vi "Periodic Tasks.vi"(8 "error in":errorcluster) -> ()   [LabVIEW 2020]
doc: "This VI runs in parallel to other tasks. It can contain as many user-defined periodic loops as you need. These can carry out PID or other sorts of timed response."
uses:
  <vilib>/Rock Robotics/WPI/DriverStation/WPI_DriverStationRobotMode2.ctl
  <vilib>/Rock Robotics/WPI/ThirdParty/Phoenix-LabVIEW/Motor Controller/Controls/CTRE_Phoenix_MotorControl_ControlMode.ctl
  <vilib>/Rock Robotics/WPI/Joystick/XBox Axes Indexer.ctl
  <vilib>/Rock Robotics/WPI/Utilities/WPI_GetSetVariantRefNum.vi
  Robot Global Data.vi
  <vilib>/Rock Robotics/Network Tables/NT Read Number.vi
  <vilib>/Rock Robotics/WPI/ThirdParty/Phoenix-LabVIEW/Motor Controller/Get/CTRE_Phoenix_MotorController_GetSelectedSensorData.vi
  <vilib>/Rock Robotics/Network Tables/NT Write Number.vi
  <vilib>/Rock Robotics/WPI/ThirdParty/Phoenix-LabVIEW/Pigeon IMU/CTRE_PigeonIMU_GetYPR.vi
  <vilib>/ptbypt/NI_PtbyPt.lvlib
panel:
  out "Drive Loop Speed":u32=37
  in  "Drive wait":u32=25
  in  "Sensor wait":u32=25
  out "Sensor Loop Speed":u32=26
  in  "Joystick wait":u32=25
  out "Joystick Loop Speed":u32=28
  in  "Rot Pt X":dbl format="%#_13g"
  in  "Rot Pt Y":dbl format="%#_13g"
  out "Robot Centric?":bool
  in  "Slow Drive Speed %":dbl=0.75
  in  "Z-axis rate modifier":dbl=0.7 format="%#_13g"
  out "Go Slow?":bool
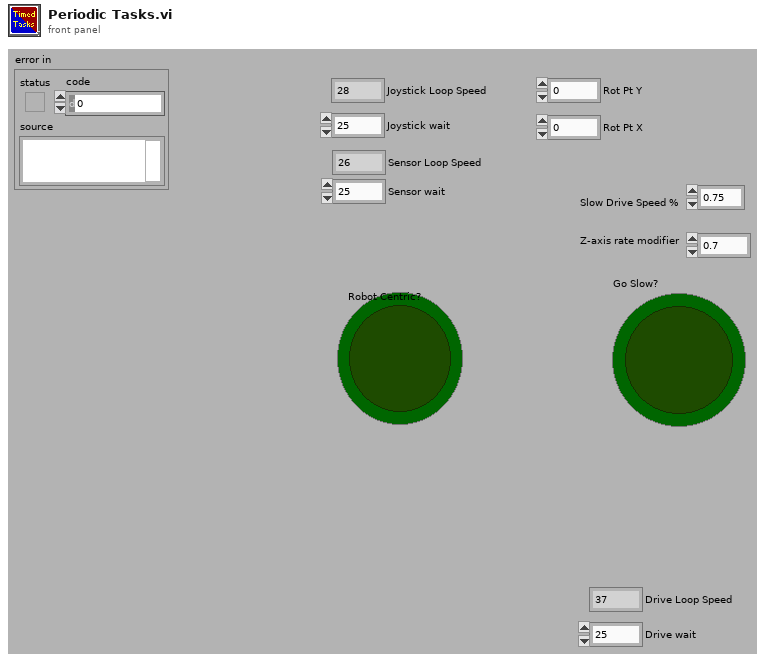
[diagram p1: front panel]
types:
  T1 = typedef "WPI_MotorControlDeviceRef.ctl" = cluster{"DeviceStatus":errorcluster, "Type":T2, "PWM":cluster{"PWM Channel":T3, "DeadBand":T4}, "CAN":cluster{"Device Number":u8, "SetOutput VI Ref":variant, "GetOutput VI Ref":variant, "Enable VI Ref":variant, "Disable VI Ref":variant, "Data":variant}, "Invert":bool, "DIO PWM":cluster{"PWM \"Enable\" Channel":T3, "DIOChannel":T5, "PWM Rate":dbl}}
  T2 = typedef "WPI_MotorControlType.ctl" = enum16{"PWM", "CAN", "DIO PWM"}
  T3 = typedef "FPGA_DIOPWMChannel.ctl" = enum8{"PWM 0", "PWM 1", "PWM 2", "PWM 3", "PWM 4", "PWM 5", "PWM 6", "PWM 7", "PWM 8", "PWM 9", "PWM MXP 0", "PWM MXP 1", "PWM MXP 2", "PWM MXP 3", "PWM MXP 4", "PWM MXP 5", "PWM MXP 6", "PWM MXP 7", "PWM MXP 8", "PWM MXP 9", "Invalid"}
  T4 = typedef "WPI_PWMDeadband.ctl" = cluster{"Name":string, "maxPositivePwm":i32, "minPositivePwm":i32, "centerPwm":i32, "maxNegativePwm":i32, "minNegativePwm":i32, "angularRange":u16}
  T5 = typedef "FPGA_DIOChannel.ctl" = enum8{"DIO 0", "DIO 1", "DIO 2", "DIO 3", "DIO 4", "DIO 5", "DIO 6", "DIO 7", "DIO 8", "DIO 9", "DIO MXP 0", "DIO MXP 1", "DIO MXP 2", "DIO MXP 3", "DIO MXP 4", "DIO MXP 5", "DIO MXP 6", "DIO MXP 7", "DIO MXP 8", "DIO MXP 9", "DIO MXP 10", "DIO MXP 11", "DIO MXP 12", "DIO MXP 13", "DIO MXP 14", "DIO MXP 15", "SPI Port CS1", "SPI Port CS2", "SPI Port CS3", "SPI Port MISO", "SPI Port MOSI", "Invalid"}
  T6 = typedef "WPI_JoystickDevRef.ctl" = cluster{"Device":T7}
  T7 = typedef "WPI_JoystickDeviceEnum.ctl" = enum16{"USB 0", "USB 1", "USB 2", "USB 3", "USB 4", "USB 5"}
  T8 = typedef "XBox Axes Indexer.ctl" = enum16{"Left X", "Left Y", "Left Trigger", "Right Trigger", "Right X", "Right Y"}
  T9 = typedef "WPI_DriverStationRobotMode2.ctl" = enum16{"Autonomous Disabled", "Autonomous Enabled", "Teleop Disabled", "Teleop Enabled", "Disconnected", "Finish", "Test Disabled", "Test Enabled", "Emergency Stopped"}
  T10 = typedef "CTRE_Phoenix_MotorControl_ControlMode.ctl" = u16
  T11 = typedef "CTRE_PigeonIMU_DeviceRef.ctl" = cluster{"DeviceStatus":errorcluster, "Device Number":u8, "Type":T12, "Device ID":u32, "Handle":u64, "UsageFrame":u32, "Library Path":path}
  T12 = typedef "CTRE_PigeonIMU_ConnectionType.ctl" = u32
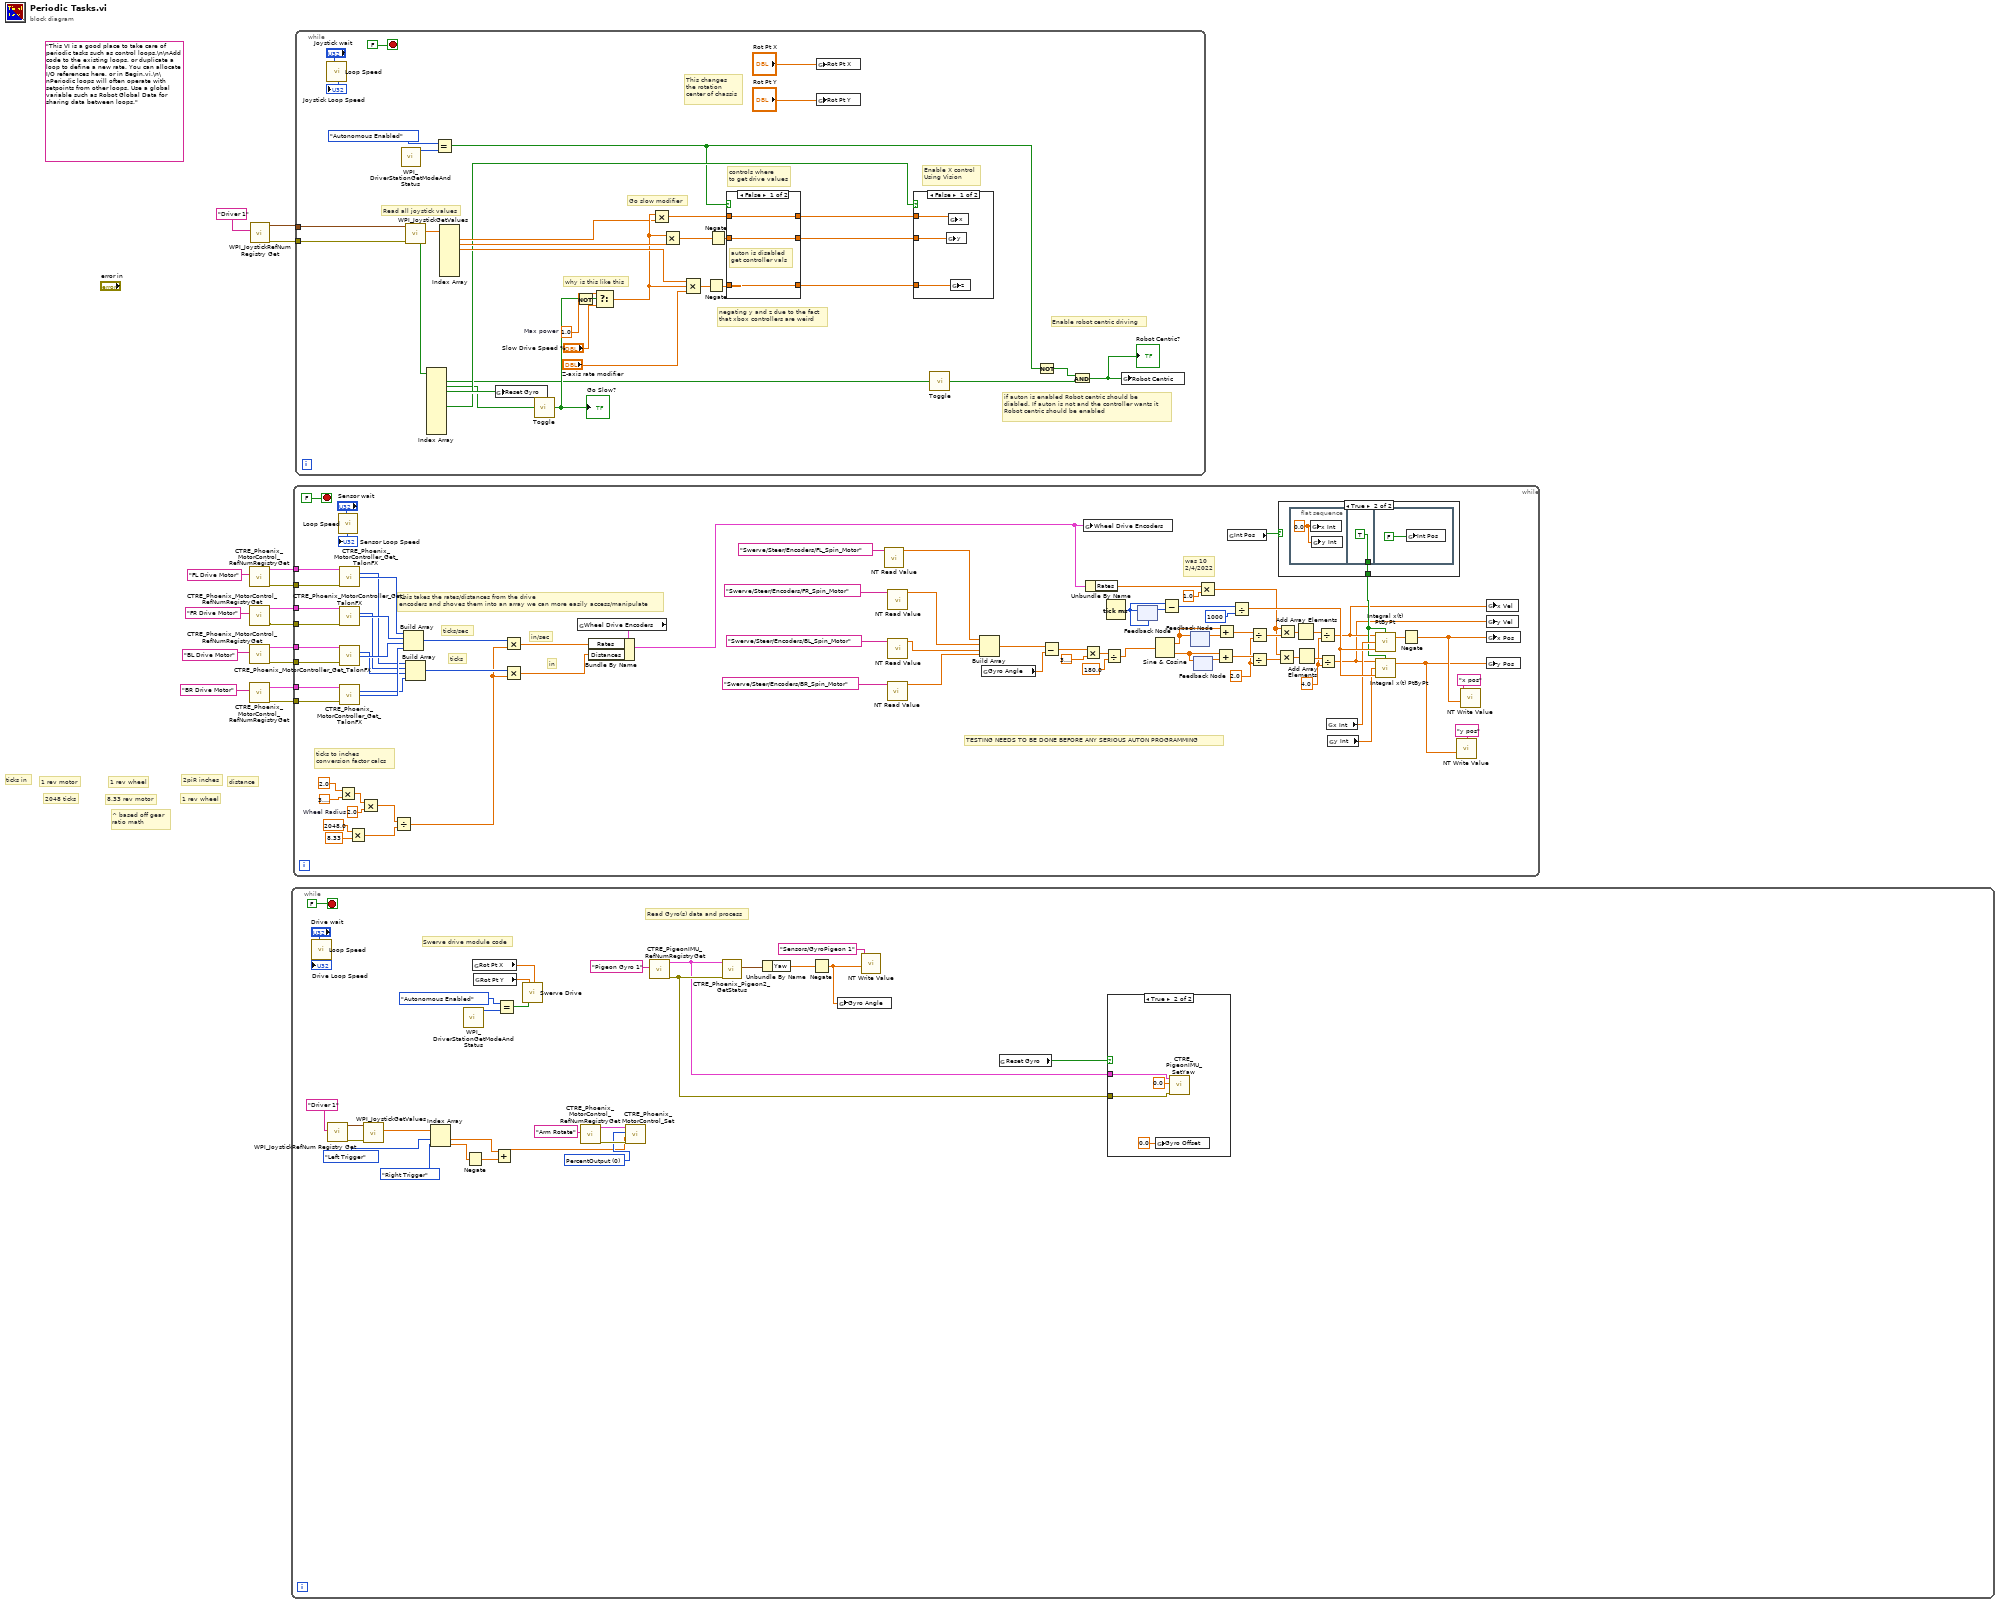
[diagram p0: block diagram]
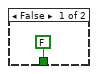
[diagram p3: hidden frame]
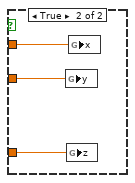
[diagram p4: hidden frame]
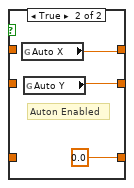
[diagram p5: hidden frame]
diagram:
  (unwired) "This VI is a good place to take care of periodic tasks such as control loops.\n\nAdd code to the existing loops, or duplicate a loop to define a new rate. You can allocate I/O references here, or in Begin.vi.\n\nPeriodic loops will often operate with setpoints from other loops. Use a global variable such as Robot Global Data for sharing data between loops."
  # "^ based off gear \nratio math"
  # "distance"
  # "2piR inches"
  # "1 rev wheel"
  # "1 rev wheel"
  # "8.33 rev motor"
  # "1 rev motor"
  # "2048 ticks"
  # "ticks in"
  n1 = call <vilib>:"CTRE_Phoenix_MotorControl_RefNumRegistryGet.vi"("refnum name"="FL Drive Motor") -> ("error out"=w7:errorcluster, "PhoenixMotorControlDevRef"=w8:T1)  [unwired: 9 in]
  n2 = call <vilib>:"CTRE_Phoenix_MotorControl_RefNumRegistryGet.vi"("refnum name"="FR Drive Motor") -> ("error out"=w5:errorcluster, "PhoenixMotorControlDevRef"=w6:T1)  [unwired: 9 in]
  n3 = call <vilib>:"CTRE_Phoenix_MotorControl_RefNumRegistryGet.vi"("refnum name"="BL Drive Motor") -> ("error out"=w3:errorcluster, "PhoenixMotorControlDevRef"=w4:T1)  [unwired: 9 in]
  n4 = call <vilib>:"CTRE_Phoenix_MotorControl_RefNumRegistryGet.vi"("refnum name"="BR Drive Motor") -> ("error out"=w1:errorcluster, "PhoenixMotorControlDevRef"=w2:T1)  [unwired: 9 in]
  n5 = call <vilib>:"WPI_JoystickRefNum Registry Get.vi"("refnum name"="Driver 1") -> ("error out"=w13:errorcluster, "JoystickDevRef"=w14:T6)  [unwired: 1 in, 8 out]
  n6 = while {
    stop <- FALSE stop-if-true
    w22 = T10 0 items=["PercentOutput"=0, "Position"=1, "Velocity"=2, "Current"=3, "Follower"=5, "MotionProfile"=6, "MotionMagic"=7, "MotionProfileArc"=10, "Disabled"=15] ("Control Mode")
    # "Read Gyro(s) data and process"
    # "Swerve drive module code"
    n7 = call "Loop Speed.vi"("milliseconds to wait"="Drive wait") -> ("Loop Speed"=→"Drive Loop Speed":u32)
    n8 = call <vilib>:"WPI_JoystickRefNum Registry Get.vi"("refnum name"="Driver 1") -> ("error out"=w26:errorcluster, "JoystickDevRef"=w25:T6)  [unwired: 9 in]
    n9 = call <vilib>:"WPI_JoystickGetValues.vi"("error in (no error)"=w26, "JoystickDevRef"=w25) -> ("Axes"=w24:dbl[])  [unwired: 5 in, 4 out]
    n10 = Index Array(array=w24, index #1=XBox_Axes_Indexer."Left Trigger" ("XBox Axes"), index #2=XBox_Axes_Indexer."Right Trigger" ("XBox Axes")) -> (element #1=w18:dbl, element #2=w20:dbl)
    n11 = call <vilib>:"WPI_DriverStationGetModeAndStatus.vi"() -> ("Robot Mode"=w39:T9)  [unwired: 10 in, 1 out]
    n12 = Negate(x=w20) -> (-x=w19:dbl)
    n13 = global read "Robot Global Data.vi" "Rot Pt X"() -> (w41:dbl)
    n14 = global read "Robot Global Data.vi" "Rot Pt Y"() -> (w40:dbl)
    n15 = Add(x=w18, y=w19) -> (x+y=w17:dbl)
    n16 = Equal?(x=WPI_DriverStationRobotMode2."Autonomous Enabled", y=w39) -> (x = y?=w42:bool)
    n17 = call "Swerve Drive.vi"("Rot. Point X"=w41, "Auto Controls"=w42, "Rot. Point Y"=w40) -> ()  [unwired: 9 in]
    n18 = call <vilib>:"CTRE_Phoenix_MotorControl_RefNumRegistryGet.vi"("refnum name"="Arm Rotate") -> ("error out"=w29:errorcluster, "PhoenixMotorControlDevRef"=w28:T1)  [unwired: 9 in]
    n19 = call <vilib>:"CTRE_Phoenix_MotorControl_Set.vi"("error in (no error)"=w29, "Output"=w17, "Control Mode"=w22, "PhoenixMotorControlDevRef"=w28) -> ()  [unwired: 6 in, 2 out]
    n20 = call <vilib>:"CTRE_PigeonIMU_RefNumRegistryGet.vi"("refnum name"="Pigeon Gyro 1") -> ("error out"=w32:errorcluster, "PigeonIMUDevRef"=w31:T11)  [unwired: 9 in]
    n21 = call-poly <vilib>:"CTRE_Phoenix_Pigeon2_GetStatus.vi"("error in (no error)"=w32, "PigeonIMUDevRef"=w31) -> ("Yaw Pitch Roll"=w36:cluster{"Yaw":dbl, "Pitch":dbl, "Roll":dbl})  [unwired: 7 in, 2 out]
    n22 = Unbundle By Name(w36) -> ("Yaw"=w37:dbl)
    n23 = Negate(x=w37) -> (-x=w30:dbl)
    n24 = global write "Robot Global Data.vi" "Gyro Angle"(w30) -> ()
    n25 = call-poly <vilib>:"NT Write Value.vi"("value"=w30, "name"="Sensors/GyroPigeon 1" ("Name")) -> ()  [unwired: 9 in, 1 out]
    n26 = global read "Robot Global Data.vi" "Reset Gyro"() -> (w33:bool)
    n27 = case shown="True" w33 {
      tunnel: w32 -> [_ w47]
      tunnel: w31 -> [_ w46]
      frame False {
      }
      frame True {
        n28 = global write "Robot Global Data.vi" "Gyro Offset"(0.0 ("Gyro Offset")) -> ()
        n29 = call <vilib>:"CTRE_PigeonIMU_SetYaw.vi"("error in (no error)"=w47, "Value"=0.0, "PigeonIMUDevRef"=w46) -> ()  [unwired: 7 in, 2 out]
      }
    }
  }
  n30 = while {
    tunnel: w8 -> [w80]
    tunnel: w7 -> [w79]
    tunnel: w6 -> [w78]
    tunnel: w5 -> [w77]
    tunnel: w4 -> [w76]
    tunnel: w3 -> [w75]
    tunnel: w2 -> [w74]
    tunnel: w1 -> [w73]
    stop <- FALSE stop-if-true
    w66 = 2.0  # Wheel Radius
    w90 = 4.0 ("y")
    w115 = 2.0
    # "TESTING NEEDS TO BE DONE BEFORE ANY SERIOUS AUTON PROGRAMMING"
    # "was 10 \n2/4/2022"
    # "ticks to inches \nconversion factor calcs"
    # "in/sec"
    # "in"
    # "ticks"
    # "ticks/sec"
    # "This takes the rates/distances from the drive \nencoders and shoves them into an array we can more easily access/manipulate"
    n31 = call "Loop Speed.vi"("milliseconds to wait"="Sensor wait") -> ("Loop Speed"=→"Sensor Loop Speed":u32)
    n32 = Multiply(x=2.0, y=3.141592653589793) -> (x*y=w67:dbl)
    n33 = call-poly <vilib>:"CTRE_Phoenix_MotorController_Get_TalonFX.vi"("PhoenixMotorControlDevRef"=w80, "error in"=w79) -> ("Position (Raw Sensor Units)"=w95:i32, "Velocity (Raw Sensor Units per 100 ms)"=w105:i32)  [unwired: 10 in, 2 out]
    n34 = call-poly <vilib>:"CTRE_Phoenix_MotorController_Get_TalonFX.vi"("PhoenixMotorControlDevRef"=w78, "error in"=w77) -> ("Position (Raw Sensor Units)"=w101:i32, "Velocity (Raw Sensor Units per 100 ms)"=w104:i32)  [unwired: 10 in, 2 out]
    n35 = call-poly <vilib>:"CTRE_Phoenix_MotorController_Get_TalonFX.vi"("PhoenixMotorControlDevRef"=w76, "error in"=w75) -> ("Position (Raw Sensor Units)"=w100:i32, "Velocity (Raw Sensor Units per 100 ms)"=w103:i32)  [unwired: 10 in, 2 out]
    n36 = call-poly <vilib>:"CTRE_Phoenix_MotorController_Get_TalonFX.vi"("PhoenixMotorControlDevRef"=w74, "error in"=w73) -> ("Position (Raw Sensor Units)"=w99:i32, "Velocity (Raw Sensor Units per 100 ms)"=w102:i32)  [unwired: 10 in, 2 out]
    n37 = Multiply(x=2048.0, y=8.33) -> (x*y=w64:dbl)
    n38 = Multiply(x=w67, y=w66) -> (x*y=w65:dbl)
    n39 = Divide(x=w65, y=w64) -> (x/y=w59:dbl)
    n40 = Build Array(w105, w104, w103, w102) -> (w60:i32[])
    n41 = Build Array(w95, w101, w100, w99) -> (w62:i32[])
    n42 = Multiply(x=w60, y=w59) -> (x*y=w58:dbl[])
    n43 = Multiply(x=w62, y=w59) -> (x*y=w61:dbl[])
    n44 = global read "Robot Global Data.vi" "Wheel Drive Encoders"() -> (w98:cluster{"Rates":dbl[], "Distances":dbl[]})
    n45 = Bundle By Name(cluster=w98, "Rates"=w58, "Distances"=w61) -> (w72:cluster{"Rates":dbl[], "Distances":dbl[]})
    n46 = call-poly <vilib>:"NT Read Value.vi"("name"="Swerve/Steer/Encoders/FL_Spin_Motor") -> ("value"=w126:dbl)  [unwired: 8 in, 2 out]
    n47 = call-poly <vilib>:"NT Read Value.vi"("name"="Swerve/Steer/Encoders/BR_Spin_Motor") -> ("value"=w123:dbl)  [unwired: 8 in, 2 out]
    n48 = call-poly <vilib>:"NT Read Value.vi"("name"="Swerve/Steer/Encoders/FR_Spin_Motor") -> ("value"=w125:dbl)  [unwired: 8 in, 2 out]
    n49 = call-poly <vilib>:"NT Read Value.vi"("name"="Swerve/Steer/Encoders/BL_Spin_Motor") -> ("value"=w124:dbl)  [unwired: 8 in, 2 out]
    n50 = Build Array(w126, w125, w124, w123) -> (w122:dbl[])
    n51 = global read "Robot Global Data.vi" "Gyro Angle"() -> (w83:dbl)
    n52 = Subtract(x=w122, y=w83) -> (x-y=w88:dbl[])
    n53 = global write "Robot Global Data.vi" "Wheel Drive Encoders"(w72) -> ()
    n54 = Multiply(x=w88, y=3.141592653589793) -> (x*y=w87:dbl[])
    n55 = Unbundle By Name(w72) -> ("Rates"=w106:dbl[])
    n56 = Divide(x=w87, y=180.0) -> (x/y=w86:dbl[])
    n57 = Tick Count (ms)() -> (millisecond timer value=w109:u32)
    n58 = feedback #1(w109) -> (w110:u32)
    n59 = feedback-in #1(w109) -> ()
    n60 = Sine & Cosine(0:w86) -> (1:w120:dbl[], 2:w118:dbl[])
    n61 = Subtract(x=w109, y=w110) -> (x-y=w108:u32)
    n62 = feedback #2() -> (w121:dbl[])  [unwired: 1 in]
    n63 = feedback-in #2(w120) -> ()
    n64 = feedback #3() -> (w119:dbl[])  [unwired: 1 in]
    n65 = feedback-in #3(w118) -> ()
    n66 = Multiply(x=w106, y=1.0) -> (x*y=w92:dbl[])
    n67 = Add(x=w118, y=w119) -> (x+y=w116:dbl[])
    n68 = Add(x=w120, y=w121) -> (x+y=w117:dbl[])
    n69 = global read "Robot Global Data.vi" "Int Pos"() -> (w57:bool)
    n70 = Divide(x=w108, y=u32 1000) -> (x/y=w94:dbl)
    n71 = Divide(x=w117, y=w115) -> (x/y=w114:dbl[])
    n72 = Divide(x=w116, y=w115) -> (x/y=w113:dbl[])
    n73 = Multiply(x=w92, y=w113) -> (x*y=w111:dbl[])
    n74 = Multiply(x=w92, y=w114) -> (x*y=w112:dbl[])
    n75 = case shown="True" w57 {
      tunnel: [FALSE w133] -> w54
      frame False {
      }
      frame True {
        n76 = flat-sequence {
          tunnel: [TRUE] -> w133
          frame #0 {
            w134 = 0.0 ("x Int")
            n77 = global write "Robot Global Data.vi" "x Int"(w134) -> ()
            n78 = global write "Robot Global Data.vi" "y Int"(w134) -> ()
          }
          frame #1 {
          }
          frame #2 {
            n79 = global write "Robot Global Data.vi" "Int Pos"(FALSE ("Int Pos")) -> ()
          }
        }
      }
    }
    n80 = Add Array Elements(numeric array=w112) -> (sum=w89:dbl)
    n81 = Add Array Elements(numeric array=w111) -> (sum=w107:dbl)
    n82 = Divide(x=w89, y=w90) -> (x/y=w53:dbl)
    n83 = Divide(x=w107, y=w90) -> (x/y=w52:dbl)
    n84 = global read "Robot Global Data.vi" "x Int"() -> (w55:dbl)
    n85 = global read "Robot Global Data.vi" "y Int"() -> (w56:dbl)
    n86 = call <vilib>:"Integral x(t) PtByPt.vi"("initialize"=w54, "dt"=w94, "initial condition"=w55, "x"=w53) -> ("integral x(t)"=w63:dbl)  [unwired: 1 out]
    n87 = call <vilib>:"Integral x(t) PtByPt.vi"("initialize"=w54, "dt"=w94, "initial condition"=w56, "x"=w52) -> ("integral x(t)"=w50:dbl)  [unwired: 1 out]
    n88 = Negate(x=w63) -> (-x=w51:dbl)
    n89 = call-poly <vilib>:"NT Write Value.vi"("value"=w50, "name"="y pos" ("Name")) -> ()  [unwired: 9 in, 1 out]
    n90 = call-poly <vilib>:"NT Write Value.vi"("value"=w51, "name"="x pos" ("Name")) -> ()  [unwired: 9 in, 1 out]
    n91 = global write "Robot Global Data.vi" "x Vel"(w53) -> ()
    n92 = global write "Robot Global Data.vi" "y Vel"(w52) -> ()
    n93 = global write "Robot Global Data.vi" "x Pos"(w51) -> ()
    n94 = global write "Robot Global Data.vi" "y Pos"(w50) -> ()
  }
  n95 = while {
    tunnel: w14 -> [w148]
    tunnel: w13 -> [w137]
    stop <- FALSE stop-if-true
    w158 = 1.0  # Max power
    # "why is this like this"
    # "negating y and z due to the fact \nthat xbox controllers are weird"
    # "if auton is enabled Robot centric should be \ndiabled. If auton is not and the controller wants it \nRobot centric should be enabled"
    # "controls where\nto get drive values"
    # "Enable X control\nUsing Vision"
    # "Enable robot centric driving"
    # "Go slow modifier"
    # "This changes\nthe rotation\ncenter of chassis"
    # "Read all joystick values"
    n96 = call "Loop Speed.vi"("milliseconds to wait"="Joystick wait") -> ("Loop Speed"=→"Joystick Loop Speed":u32)
    n97 = call <vilib>:"WPI_DriverStationGetModeAndStatus.vi"() -> ("Robot Mode"=w151:T9)  [unwired: 10 in, 1 out]
    n98 = call <vilib>:"WPI_JoystickGetValues.vi"("error in (no error)"=w137, "JoystickDevRef"=w148) -> ("Buttons"=w168:bool[], "Axes"=w169:dbl[])  [unwired: 5 in, 3 out]
    n99 = Index Array(array=w168) -> (element #1=w142:bool, element #2=w143:bool, element #3=w166:bool, element #6=w147:bool)  [unwired: 11 in, 7 out]
    n100 = Equal?(x=WPI_DriverStationRobotMode2."Autonomous Enabled", y=w151) -> (x = y?=w141:bool)
    n101 = Index Array(array=w169) -> (element #1=w152:dbl, element #2=w167:dbl, element #5=w162:dbl)  [unwired: 8 in, 5 out]
    n102 = global write "Robot Global Data.vi" "Reset Gyro"(w166) -> ()
    n103 = call "Toggle.vi"("Input"=w143) -> ("Output"=w144:bool)
    "Go Slow?" <- w144
    n104 = Not(x=w144) -> (.not. x?=w157:bool)
    n105 = Select(t=w158, s=w157, f="Slow Drive Speed %") -> (s? t:f=w155:dbl)
    n106 = Multiply(x=w155, y=w152) -> (x*y=w160:dbl)
    n107 = Multiply(x=w155, y=w167) -> (x*y=w159:dbl)
    n108 = Compound Arithmetic op=MULTIPLY(w162, w155, "Z-axis rate modifier") -> (w156:dbl)
    n109 = Negate(x=w156) -> (-x=w164:dbl)
    n110 = Negate(x=w159) -> (-x=w165:dbl)
    n111 = case shown="False" w141 {
      tunnel: w165 -> [w180 _]
      tunnel: w160 -> [w179 _]
      tunnel: w164 -> [w181 _]
      tunnel: [w179 w182] -> w153
      tunnel: [w180 w183] -> w149
      tunnel: [w181 0.0] -> w154
      frame False {
        # "auton is disabled\nget controller vals"
      }
      frame True {
        # "Auton Enabled"
        n112 = global read "Robot Global Data.vi" "Auto X"() -> (w182:dbl)
        n113 = global read "Robot Global Data.vi" "Auto Y"() -> (w183:dbl)
      }
    }
    n114 = global write "Robot Global Data.vi" "Rot Pt X"("Rot Pt X") -> ()
    n115 = global write "Robot Global Data.vi" "Rot Pt Y"("Rot Pt Y") -> ()
    n116 = case shown="False" w147 {
      tunnel: w153 -> [w173 w177]
      tunnel: w154 -> [w175 w178]
      tunnel: w149 -> [w174 w176]
      frame False {
        n117 = global write "Robot Global Data.vi" "y"(w174) -> ()
        n118 = global write "Robot Global Data.vi" "x"(w173) -> ()
        n119 = global write "Robot Global Data.vi" "z"(w175) -> ()
      }
      frame True {
        n120 = global write "Robot Global Data.vi" "y"(w176) -> ()
        n121 = global write "Robot Global Data.vi" "z"(w178) -> ()
        n122 = global write "Robot Global Data.vi" "x"(w177) -> ()
      }
    }
    n123 = call "Toggle.vi"("Input"=w142) -> ("Output"=w139:bool)
    n124 = Not(x=w141) -> (.not. x?=w140:bool)
    n125 = And(x=w140, y=w139) -> (x .and. y?=w138:bool)
    "Robot Centric?" <- w138
    n126 = global write "Robot Global Data.vi" "Robot Centric"(w138) -> ()
  }
